vi "Read Config.vi"(8 "error in (no error)":errorcluster, 11 "ConfigurationFileName":string="SerialConfig.xml") -> (0 "error out":errorcluster, 3 "DeviceList":T1[](array[typedef]))   [LabVIEW 2010, in "MonitorServer.lvlib"]
doc: "Use this template to build a VI to use as a subVI."
uses:
  MonitorServer.lvlib
  Serial Config.ctl
  <vilib>/Utility/xml.llb/Read From XML File(string).vi
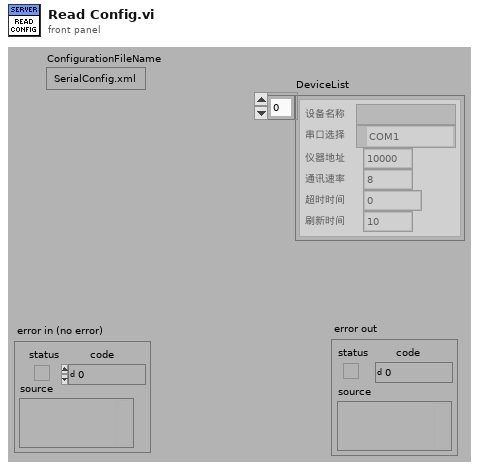
[diagram p1: front panel]
types:
  T1 = typedef "MonitorServer.lvlib/Serial Config.ctl" = cluster{"设备名称":string, "串口选择":refnum<visa-resource-name>, "仪器地址":u32, "通讯速率":u32, "超时时间":u32, "刷新时间":dbl}
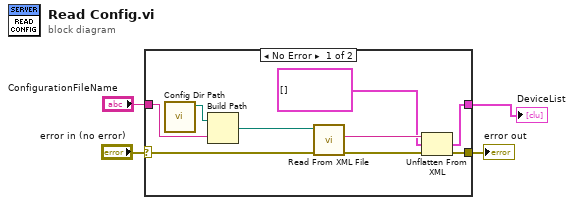
[diagram p0: block diagram]
diagram:
  n1 = case shown="No Error" "error in (no error)" {
    selector: "error in (no error)" -> [w12 w14]
    tunnel: [w7 w14] -> w2
    tunnel: "ConfigurationFileName" -> [w10 _]
    tunnel: [w6 _] -> w1
    frame No Error {
      n2 = call "Config Dir Path.vi"() -> ("App.Dir"=w8:path)  [unwired: 11 in]
      n3 = Build Path(base path=w8, name or relative path=w10) -> (appended path=w9:path)
      n4 = call-poly <vilib>:"Read From XML File.vi"("error in (no error)"=w12, "XML File Path"=w9) -> ("error out"=w11:errorcluster, "XML Elements"=w13:string)  [unwired: 7 in, 1 out]
      n5 = Unflatten From XML(xml string=w13, type=T1[] [], error in (no error)=w11) -> (value=w6:T1[], error out=w7:errorcluster)
    }
    frame Error {
    }
  }
  "error out" <- w2
  "DeviceList" <- w1
